vi "Multiple U3 with Multiple AIN Loops.vi"() -> ()   [LabVIEW 2021]
panel:
  out "Error Index":i32
  out "error":errorcluster
  in  "Device Addresses":i32[](array[numeric])=[2, 3]
  in  "Collect First n Channels From Each":u32=3
  out "Readings":dbl[](array[numeric]) format="%.6f"
  in  "stop":bool
  in  "Interval (ms)":u32=500
  out "Error Message":string
  # "The examples \"Multiple U3 with Multiple\nAIN Parallel.vi\" and \"Multiple U3 Efunction\nLoop Example.vi\" show a basic technique of\ntalking to multiple devices in parallel, but\nthese example shows a more advanced\narray/loop technique that would easily\nextend to lots of devices."
  # "An address can be a Local ID or\nSerial Number.\n\nTo remove an element, right-click\non it, select Data Operations =>\nRemove Element.\n\nTo empty an array, right-click\nnear the edge, select Data\nOperations => Empty Array.\n\nOther useful operations:  From the\nOperate menu are \"Make Current\nValues Default\" and \"Reinitialize\nTo Default\"."
  # "This index corresponds\nto the Device Addresses\narray."
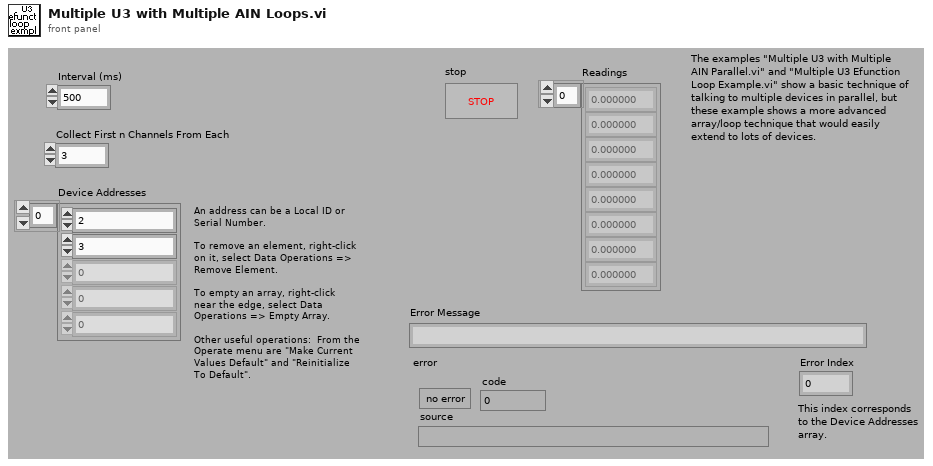
[diagram p1: front panel]
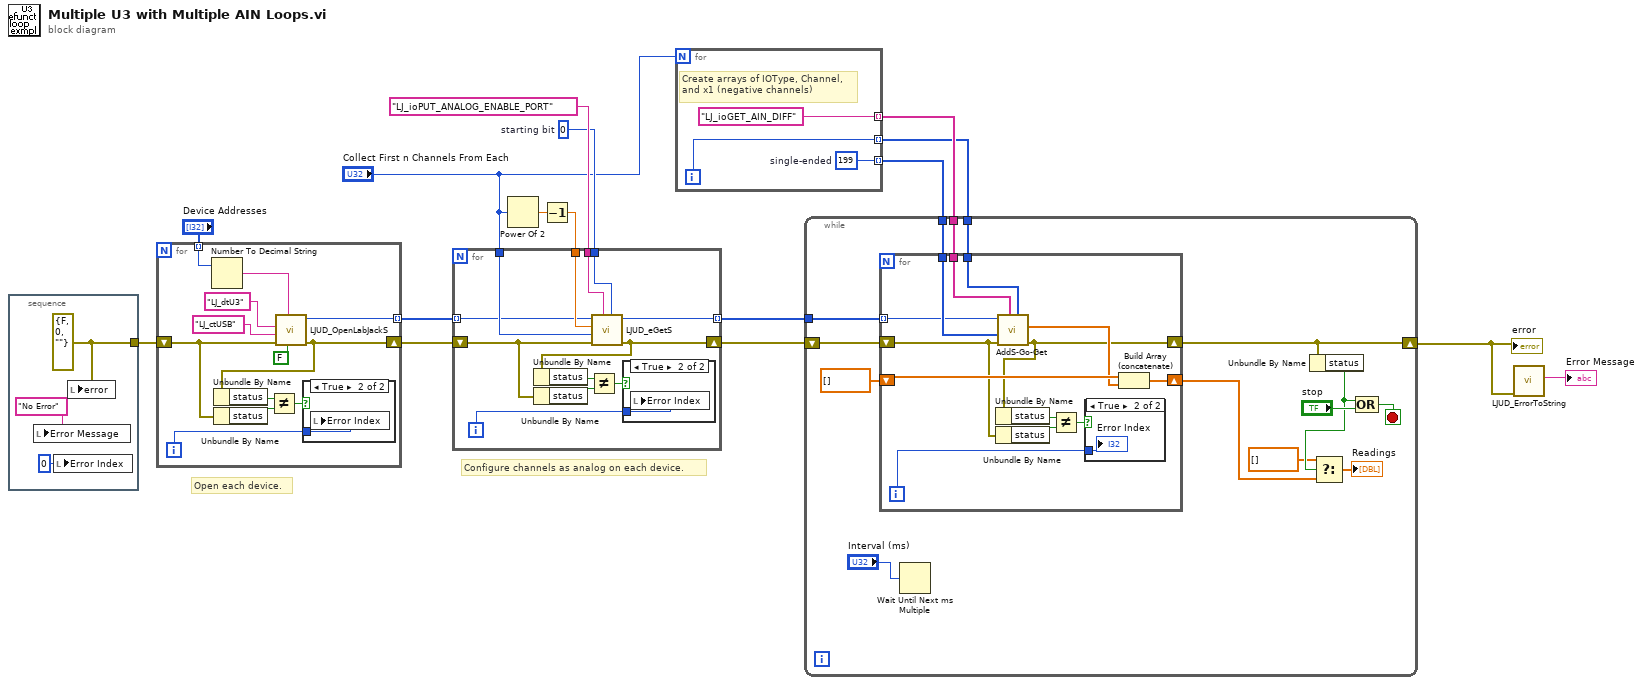
[diagram p0: block diagram]
diagram:
  w11 = 0  # starting bit
  # "Open each device."
  # "Configure channels as analog on each device."
  n1 = stacked-sequence {
    tunnel: [w19] -> w5
    frame #0 {
      w19 = errorcluster {"status"=FALSE, "code"=0, "source"=""} ("error out")
      n2 = local write "Error Message"("No Error" ("Error Message")) -> ()
      n3 = local write "Error Index"(0 ("Error Index")) -> ()
      n4 = local write "error"(w19) -> ()
    }
  }
  n5 = for {
    shift-right: [w21] -> w2
    shift-left: w5 -> [w20]
    tunnel: "Device Addresses" -> [w27] mode=indexing
    tunnel: [w26] -> w4 mode=indexing
    i -> [w22]
    n6 = Number To Decimal String(number=w27) -> (decimal integer string=w28:string)  [unwired: 1 in]
    n7 = Unbundle By Name(w20) -> ("status"=w24:bool)
    n8 = call "LJUD_OpenLabJackS.vi"("FirstFound"=FALSE, "Address"=w28, "error in"=w20, "ConnectionType"="LJ_ctUSB", "DeviceType"="LJ_dtU3") -> ("error out"=w21:errorcluster, "Handle"=w26:i32)  [unwired: 4 in, 1 out]
    n9 = Unbundle By Name(w21) -> ("status"=w25:bool)
    n10 = Not Equal?(x=w25, y=w24) -> (x != y?=w23:bool)
    n11 = case shown="True" w23 {
      tunnel: w22 -> [_ w32]
      frame False {
      }
      frame True {
        n12 = local write "Error Index"(w32) -> ()
      }
    }
  }
  n13 = Power Of 2(x="Collect First n Channels From Each") -> (2^x=w8:dbl)
  n14 = Decrement(x=w8) -> (x-1=w7:dbl)
  n15 = for {
    tunnel: "LJ_ioPUT_ANALOG_ENABLE_PORT" ("IOType") -> [w44]
    tunnel: w11 -> [w43]
    tunnel: "Collect First n Channels From Each" -> [w42]
    tunnel: w7 -> [w41]
    shift-right: [w35] -> w16
    shift-left: w2 -> [w34]
    tunnel: w4 -> [w40] mode=indexing
    tunnel: [w39] -> w3 mode=indexing
    i -> [w33]
    n16 = Unbundle By Name(w34) -> ("status"=w37:bool)
    n17 = call "LJUD_eGetS.vi"("Channel"=w43, "IOType"=w44, "error in"=w34, "x1"=w42, "Value Write"=w41, "Handle In"=w40) -> ("error out"=w35:errorcluster, "Handle Out"=w39:i32)  [unwired: 3 in, 1 out]
    n18 = Unbundle By Name(w35) -> ("status"=w36:bool)
    n19 = Not Equal?(x=w36, y=w37) -> (x != y?=w38:bool)
    n20 = case shown="True" w38 {
      tunnel: w33 -> [_ w45]
      frame False {
      }
      frame True {
        n21 = local write "Error Index"(w45) -> ()
      }
    }
  }
  n22 = for {
    N: "Collect First n Channels From Each" -> [_]
    tunnel: ["LJ_ioGET_AIN_DIFF" ("IOType")] -> w15 mode=indexing
    tunnel: [w47] -> w14 mode=indexing
    tunnel: [w46] -> w13 mode=indexing
    i -> [w47]
    w46 = 199  # single-ended
    # "Create arrays of IOType, Channel,\nand x1 (negative channels)"
  }
  n23 = while {
    tunnel: w13 -> [w56]
    tunnel: w14 -> [w57]
    tunnel: w15 -> [w58]
    shift-left: w16 -> [w53]
    shift-right: [w60] -> w1
    tunnel: w3 -> [w55]
    stop <- w59 stop-if-true
    n24 = for {
      tunnel: w58 -> [w75]
      tunnel: w57 -> [w74]
      tunnel: w56 -> [w73]
      tunnel: w55 -> [w72] mode=indexing
      shift-right: [w69] -> w51
      shift-left: dbl[] [] -> [w71]
      shift-right: [w65] -> w60
      shift-left: w53 -> [w66]
      i -> [w63]
      n25 = Unbundle By Name(w66) -> ("status"=w67:bool)
      n26 = call "AddS-Go-Get.vi"("Channels"=w74, "IOTypes"=w75, "error in"=w66, "x1"=w73, "Handle In"=w72) -> ("error out"=w65:errorcluster, "Values Read"=w70:dbl[])  [unwired: 4 in, 1 out]
      n27 = Unbundle By Name(w65) -> ("status"=w68:bool)
      n28 = Not Equal?(x=w68, y=w67) -> (x != y?=w64:bool)
      n29 = case shown="True" w64 {
        tunnel: w63 -> [_ w76]
        frame False {
        }
        frame True {
          "Error Index" <- w76
        }
      }
      n30 = Build Array (concatenate)(w71, w70) -> (w69:dbl[])
    }
    n31 = Wait Until Next ms Multiple(millisecond multiple="Interval (ms)") -> ()  [unwired: 1 out]
    n32 = Unbundle By Name(w60) -> ("status"=w52:bool)
    n33 = Select(t=dbl[] [], s=w52, f=w51) -> (s? t:f=→"Readings":dbl[])
    n34 = Compound Arithmetic op=OR(w52, "stop") -> (w59:bool)
  }
  "error" <- w1
  n35 = call "LJUD_ErrorToString.vi"("error in"=w1) -> ("String"=→"Error Message":string)  [unwired: 10 in]
